vi "DataLog Read Last Number.vi"(7 "tag":string, 9 "tag index in (name lookup)":i32=-1, 11 "error in (no error)":errorcluster) -> (4 "number":dbl format="%#_7g", 6 "time":dbl format="%<%H:%M:%S%2u\n%Y/%m/%d>T", 10 "tag index out":i32, 15 "error out":errorcluster)   [LabVIEW 2012]
doc: "Reads the last-written number (the current value) from a number tag of the live database. This is a convenience wrapper around the \"Tag Buffers\" object which provides a more complete set of methods for reading values from a tag's buffer."
uses:
  typedefs/t_DataLog Tag Buffers Methods.ctl
  typedefs/t_DataLog Tag Hash Methods.ctl
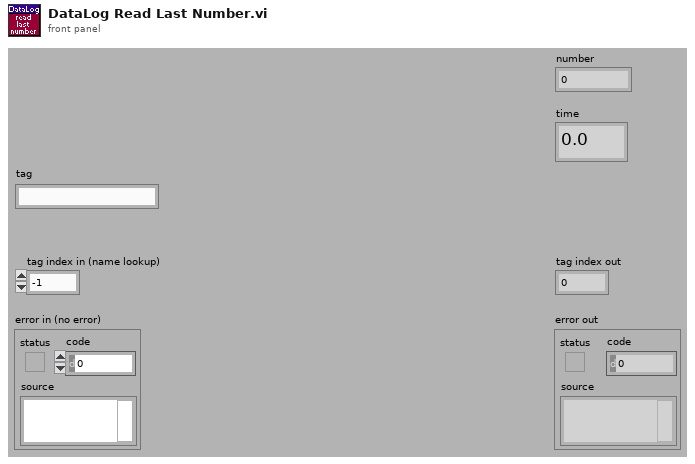
[diagram p1: front panel]
types:
  T1 = typedef "t_DataLog Tag Buffers Methods.ctl" = enum16{"initialize", "inert", "write", "read", "read oldest", "read last", "cleanup"}
  T2 = typedef "t_DataLog Tag Hash Methods.ctl" = enum16{"initialize", "add tag", "index tag", "lookup", "#tags", "cleanup", "write recovery", "read recovery", "delete recovery"}
  T3 = typedef "t_DataLog Point.ctl" = cluster{"time":dbl, "value":dbl}
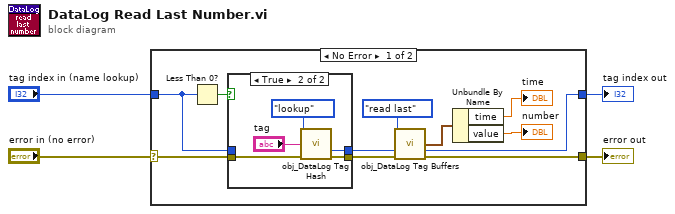
[diagram p0: block diagram]
diagram:
  n1 = case shown="No Error" "error in (no error)" {
    selector: "error in (no error)" -> [w15 w24]
    tunnel: [w13 w24] -> w3
    tunnel: "tag index in (name lookup)" -> [w9 w23]
    tunnel: [w8 w23] -> w1
    frame No Error {
      n2 = Less Than 0?(x=w9) -> (x < 0?=w10:bool)
      n3 = case shown="True" w10 {
        tunnel: w15 -> [w17 w22]
        tunnel: [w17 w20] -> w14
        tunnel: [w16 w19] -> w11
        tunnel: w9 -> [w16 _]
        frame False {
        }
        frame True {
          n4 = call "obj_DataLog Tag Hash.vi"("method"=t_DataLog_Tag_Hash_Methods."lookup", "tag in"="tag", "error in (no error)"=w22) -> ("tag index out"=w19:i32, "error out"=w20:errorcluster)  [unwired: 9 in, 2 out]
        }
      }
      n5 = call "obj_DataLog Tag Buffers.vi"("method"=t_DataLog_Tag_Buffers_Methods."read last", "tag index"=w11, "error in (no error)"=w14) -> ("point out"=w7:T3, "tag index dup"=w8:i32, "error out"=w13:errorcluster)  [unwired: 8 in, 2 out]
      n6 = Unbundle By Name(w7) -> ("time"=→"time":dbl, "value"=→"number":dbl)
    }
    frame Error {
    }
  }
  "error out" <- w3
  "tag index out" <- w1
